vi "Radau5_Sim Stop.vi"(11 "Simulation Data In":T1 {"Absolute tolerance" format="%.1e"; "Relative tolerance" format="%.1e"; "Output of T" format="%.1e"; "proposed step size" format="%.1e"; "min step size" format="%.1e"; "max step size" format="%.1e"; "final time" format="%.1e"; "step size" format="%.1e"; "initial time" format="%.1e"}) -> (0 "Stop simulation?":bool, 3 "Simulation Data Out":T1 {"Absolute tolerance" format="%.1e"; "Relative tolerance" format="%.1e"; "Output of T" format="%.1e"; "proposed step size" format="%.1e"; "min step size" format="%.1e"; "max step size" format="%.1e"; "final time" format="%.1e"; "step size" format="%.1e"; "initial time" format="%.1e"})   [LabVIEW 2020, in "NI_DAE.lvlib"]
uses:
  <vilib>/gmath/NI_DAE.lvlib
  <vilib>/gmath/dae.llb/Radau5_Simulation Data.ctl
  <vilib>/gmath/dae.llb/Radau5_Diag Eval Stage.ctl
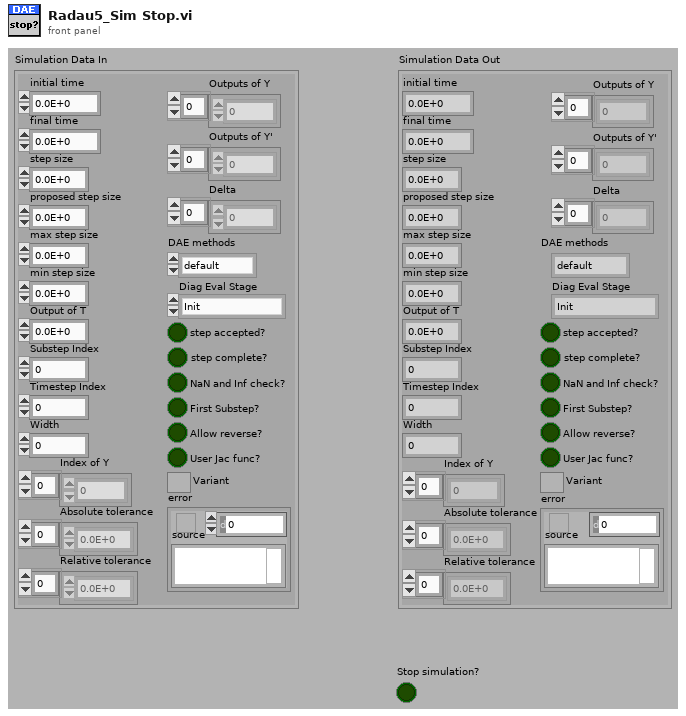
[diagram p1: front panel]
types:
  T1 = typedef "NI_DAE.lvlib/Radau5_Simulation Data.ctl" = cluster{"initial time":dbl, "final time":dbl, "step size":dbl, "proposed step size":dbl, "max step size":dbl, "min step size":dbl, "Output of T":dbl, "Substep Index":i32, "Timestep Index":i32, "Width":i32, "Absolute tolerance":dbl[], "Relative tolerance":dbl[], "Outputs of Y":dbl[], "Outputs of Y'":dbl[], "Delta":dbl[], "DAE methods":enum16{"default", "Radau IIA"}, "Diag Eval Stage":T2, "step accepted?":bool, "step complete?":bool, "NaN and Inf check?":bool, "First Substep?":bool, "Allow reverse?":bool, "error":errorcluster, "User Jac func?":bool, "Variant":variant, "Index of Y":i8[]}
  T2 = typedef "NI_DAE.lvlib/Radau5_Diag Eval Stage.ctl" = enum16{"Init", "Running", "Final", "End"}
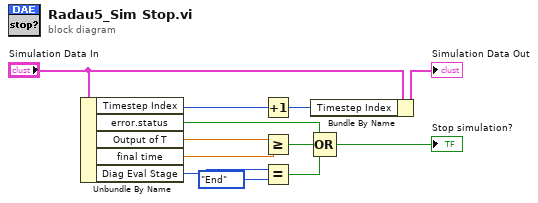
[diagram p0: block diagram]
diagram:
  n1 = Unbundle By Name("Simulation Data In") -> ("Timestep Index"=w7:i32, "error.status"=w8:bool, "Output of T"=w3:dbl, "final time"=w2:dbl, "Diag Eval Stage"=w12:T2)
  n2 = Increment(x=w7) -> (x+1=w5:i32)
  n3 = Greater Or Equal?(x=w3, y=w2) -> (x >= y?=w1:bool)
  n4 = Equal?(x=w12, y=Radau5_Diag_Eval_Stage."End" ("Diag Eval Stage")) -> (x = y?=w10:bool)
  n5 = Bundle By Name(cluster="Simulation Data In", "Timestep Index"=w5) -> (→"Simulation Data Out":T1)
  n6 = Compound Arithmetic op=OR(w8, w1, w10) -> (→"Stop simulation?":bool)
